vi "Drive at Angle.vi"(4 "end power":dbl, 6 "Begin power":dbl, 8 "error in (no error)":errorcluster, 9 "Angle":dbl, 10 "Distance":dbl, 11 "RobotDriveDevRef":T1={"DevStatus"={"status"=FALSE, "code"=0, "source"=""}, "Motors[]"=[], "Square Inputs"=FALSE, "Max Output"=1.0}) -> (0 "error out":errorcluster, 1 "power out":dbl, 3 "refnum":T1={"DevStatus"={"status"=FALSE, "code"=0, "source"=""}, "Motors[]"=[], "Square Inputs"=FALSE, "Max Output"=1.0})   [LabVIEW 2017]
uses:
  <vilib>/Rock Robotics/WPI/RobotDrive/WPI_RobotDriveDevRef.ctl
  <vilib>/Rock Robotics/WPI/MotorControl/WPI_MotorControlDeviceRef.ctl
  <vilib>/Rock Robotics/WPI/MotorControl/WPI_MotorControlType.ctl
  <vilib>/Rock Robotics/SystemInterfaces/DIO/FPGA_DIOPWMChannel.ctl
  <vilib>/Rock Robotics/WPI/PWM/WPI_PWMDeadband.ctl
  <vilib>/Rock Robotics/SystemInterfaces/DIO/FPGA_DIOChannel.ctl
  Robot Global Data.vi
  <vilib>/Rock Robotics/WPI/RobotDrive/WPI_RobotDriveArcadeDrive_Standard(NoSaturation).vi
panel:
  out "error":dbl
  out "x/y":dbl
  out "Distance Left 2":dbl format="%#_13g"
  out "rampdown":dbl format="%#_13g"
  out "Maximup":dbl format="%#_13g"
  out "rampup":dbl format="%#_13g"
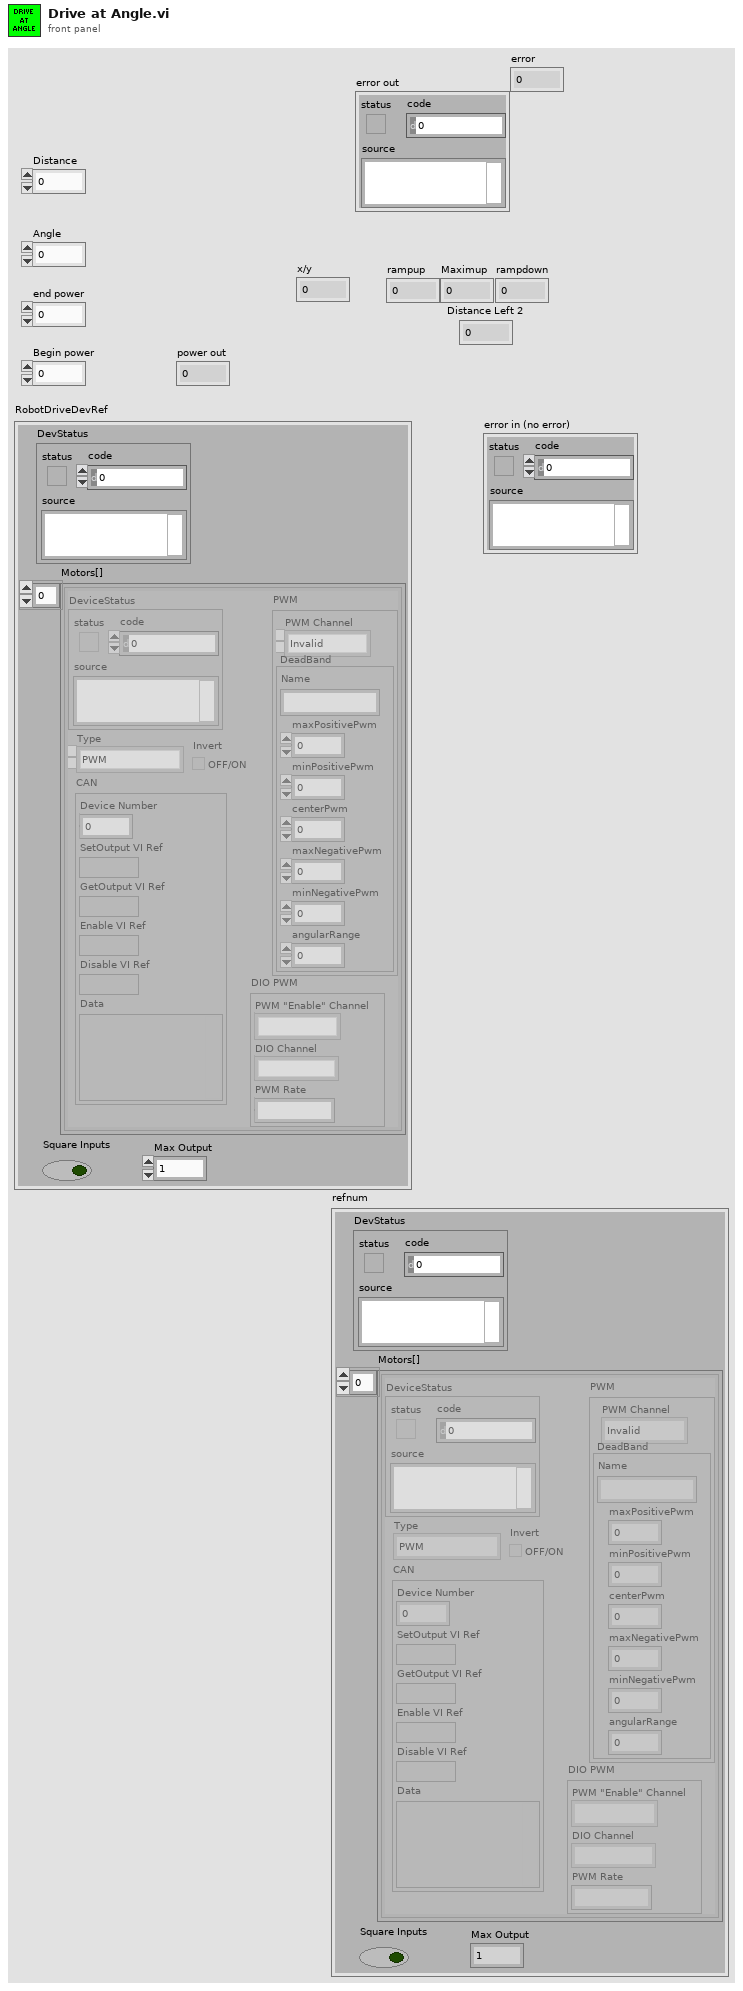
[diagram p1: front panel]
types:
  T1 = typedef "WPI_RobotDriveDevRef.ctl" = cluster{"DevStatus":errorcluster, "Motors[]":T2[], "Square Inputs":bool, "Max Output":dbl}
  T2 = typedef "WPI_MotorControlDeviceRef.ctl" = cluster{"DeviceStatus":errorcluster, "Type":T3, "PWM":cluster{"PWM Channel":T4, "DeadBand":T5}, "CAN":cluster{"Device Number":u8, "SetOutput VI Ref":variant, "GetOutput VI Ref":variant, "Enable VI Ref":variant, "Disable VI Ref":variant, "Data":variant}, "Invert":bool, "DIO PWM":cluster{"PWM \"Enable\" Channel":T4, "DIOChannel":T6, "PWM Rate":dbl}}
  T3 = typedef "WPI_MotorControlType.ctl" = enum16{"PWM", "CAN", "DIO PWM"}
  T4 = typedef "FPGA_DIOPWMChannel.ctl" = enum8{"PWM 0", "PWM 1", "PWM 2", "PWM 3", "PWM 4", "PWM 5", "PWM 6", "PWM 7", "PWM 8", "PWM 9", "PWM MXP 0", "PWM MXP 1", "PWM MXP 2", "PWM MXP 3", "PWM MXP 4", "PWM MXP 5", "PWM MXP 6", "PWM MXP 7", "PWM MXP 8", "PWM MXP 9", "Invalid"}
  T5 = typedef "WPI_PWMDeadband.ctl" = cluster{"Name":string, "maxPositivePwm":i32, "minPositivePwm":i32, "centerPwm":i32, "maxNegativePwm":i32, "minNegativePwm":i32, "angularRange":u16}
  T6 = typedef "FPGA_DIOChannel.ctl" = enum8{"DIO 0", "DIO 1", "DIO 2", "DIO 3", "DIO 4", "DIO 5", "DIO 6", "DIO 7", "DIO 8", "DIO 9", "DIO MXP 0", "DIO MXP 1", "DIO MXP 2", "DIO MXP 3", "DIO MXP 4", "DIO MXP 5", "DIO MXP 6", "DIO MXP 7", "DIO MXP 8", "DIO MXP 9", "DIO MXP 10", "DIO MXP 11", "DIO MXP 12", "DIO MXP 13", "DIO MXP 14", "DIO MXP 15", "SPI Port CS1", "SPI Port CS2", "SPI Port CS3", "SPI Port MISO", "SPI Port MOSI", "Invalid"}
  T7 = typedef "WPI_EncoderDevRef.ctl" = cluster{"DevStatus":errorcluster, "EncoderIndex":T8, "CounterIndex":T9, "DistancePerCount":dbl, "Decoding Type":T10}
  T8 = typedef "FPGA_EncoderIdx.ctl" = enum8{"Enc 0", "Enc 1", "Enc 2", "Enc 3", "Enc 4", "Enc 5", "Enc 6", "Enc 7", "Invalid"}
  T9 = typedef "FPGA_CounterCtrSystemIndex.ctl" = enum8{"Ctr 0", "Ctr 1", "Ctr 2", "Ctr 3", "Ctr 4", "Ctr 5", "Ctr 6", "Ctr 7", "Invalid"}
  T10 = typedef "WPI_EncoderType.ctl" = enum16{"1x", "2x", "4x"}
  T11 = cluster{"Yaw":dbl, "Roll":dbl, "Pitch":dbl, "Heading":dbl, "Fused Heading":dbl}
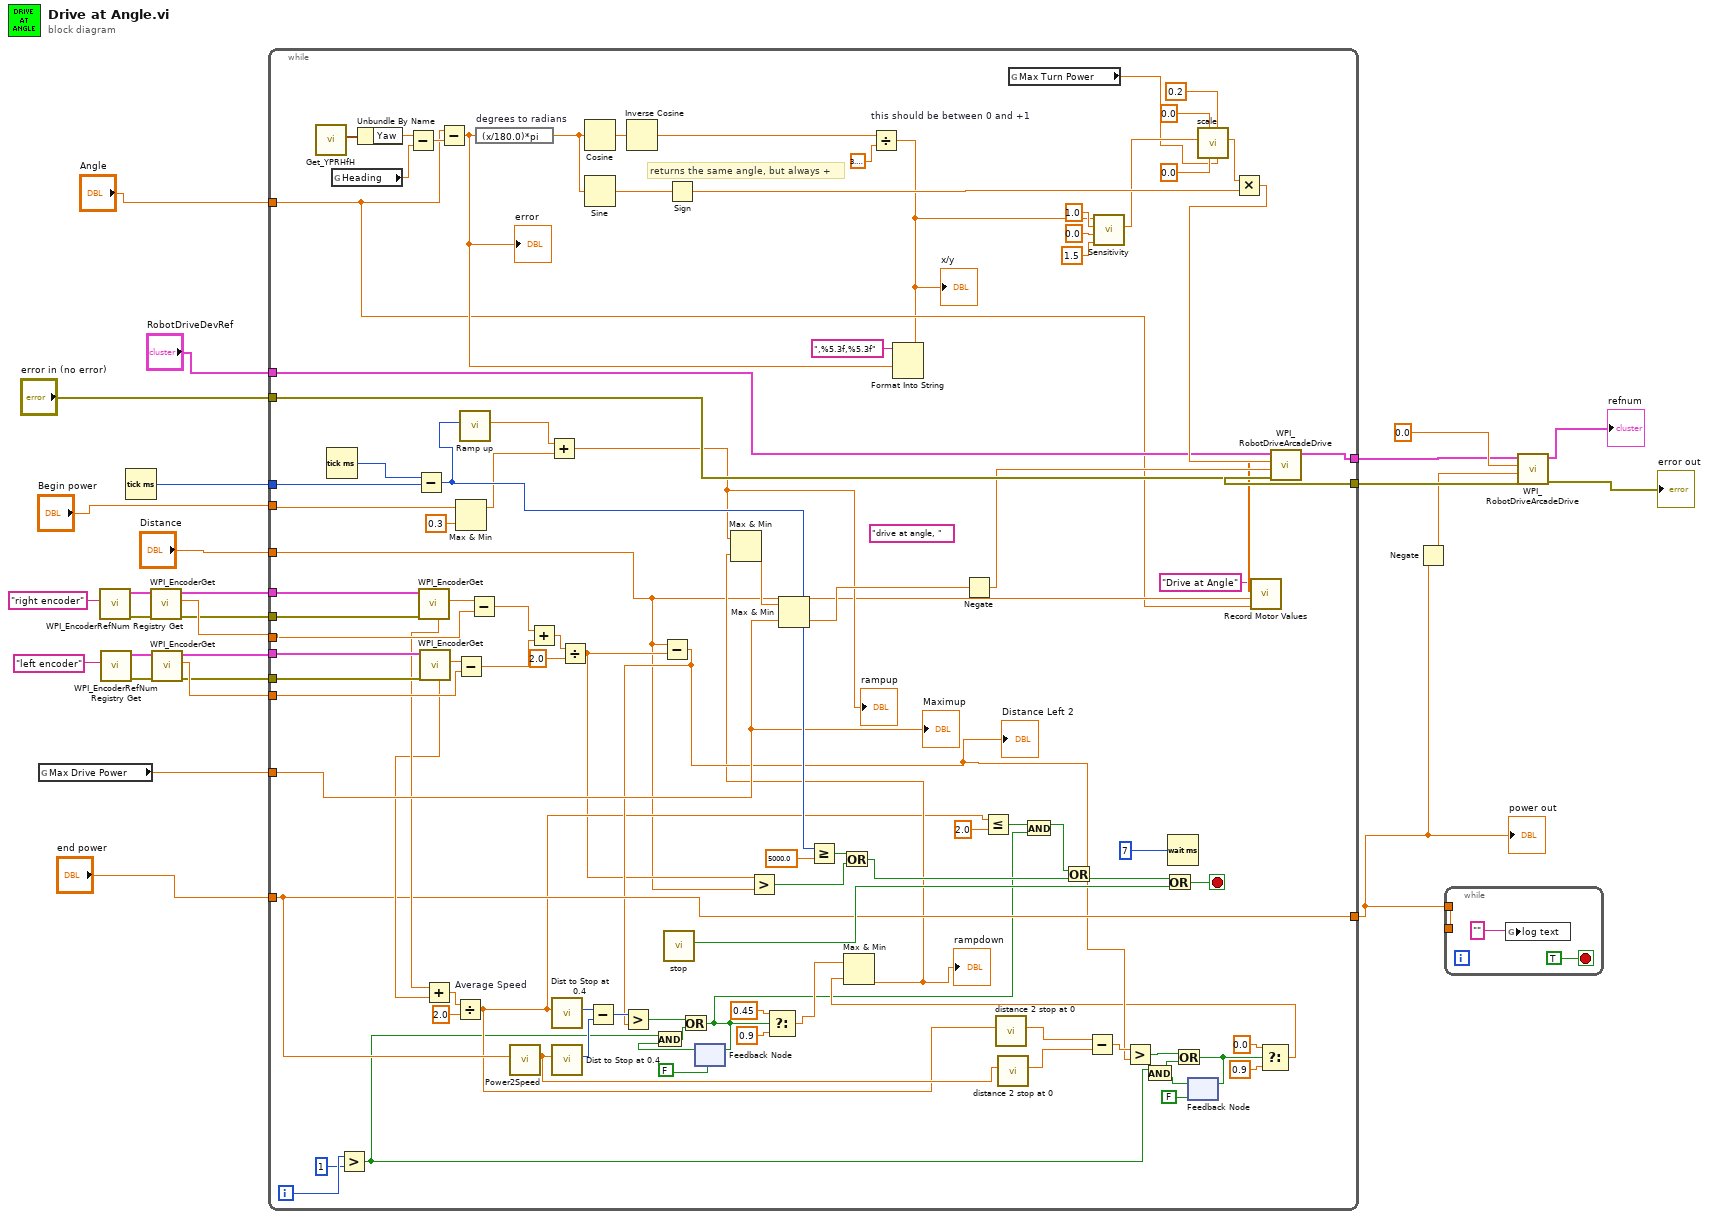
[diagram p0: block diagram]
diagram:
  n1 = global read "Robot Global Data.vi" "Max Drive Power"() -> (w3:dbl)
  n2 = call <vilib>:"WPI_EncoderRefNum Registry Get.vi"("refnum name"="right encoder") -> ("error out"=w27:errorcluster, "EncoderDevRef"=w26:T7)  [unwired: 9 in]
  n3 = call <vilib>:"WPI_EncoderRefNum Registry Get.vi"("refnum name"="left encoder") -> ("error out"=w24:errorcluster, "EncoderDevRef"=w23:T7)  [unwired: 9 in]
  n4 = Tick Count (ms)() -> (millisecond timer value=w12:u32)
  n5 = call <vilib>:"WPI_EncoderGet.vi"("error in (no error)"=w27, "EncoderDevRef"=w26) -> ("error out"=w15:errorcluster, "Distance"=w21:dbl, "EncoderDevRef"=w16:T7)  [unwired: 4 in, 3 out]
  n6 = call <vilib>:"WPI_EncoderGet.vi"("error in (no error)"=w24, "EncoderDevRef"=w23) -> ("error out"=w14:errorcluster, "Distance"=w20:dbl, "EncoderDevRef"=w13:T7)  [unwired: 4 in, 3 out]
  n7 = while {
    tunnel: "Distance" -> [w38]
    tunnel: w21 -> [w125]
    tunnel: w20 -> [w126]
    tunnel: [w124] -> w18
    tunnel: [w123] -> w17
    tunnel: w16 -> [w122]
    tunnel: w15 -> [w121]
    tunnel: w14 -> [w120]
    tunnel: w13 -> [w119]
    tunnel: w12 -> [w113]
    tunnel: [w78] -> w1
    tunnel: "Angle" -> [w37]
    tunnel: "end power" -> [w78]
    tunnel: "RobotDriveDevRef" -> [w89]
    tunnel: "error in (no error)" -> [w88]
    tunnel: "Begin power" -> [w35]
    tunnel: w3 -> [w83]
    i -> [w48]
    stop <- w91 stop-if-true
    (unwired) "drive at angle, " ("string")
    # "returns the same angle, but always +"
    n8 = call <vilib>:"Get_YPRHfH.vi"() -> ("YRPHfH"=w111:T11)  [unwired: 11 in]
    n9 = Tick Count (ms)() -> (millisecond timer value=w112:u32)
    n10 = global read "Robot Global Data.vi" "Heading"() -> (w106:dbl)
    n11 = Greater?(x=w48, y=1) -> (0:w44:bool)
    n12 = Unbundle By Name(w111) -> ("Yaw"=w107:dbl)
    n13 = Subtract(x=w107, y=w106) -> (x-y=w105:dbl)
    n14 = Subtract(x=w112, y=w113) -> (x-y=w90:u32)
    n15 = call <vilib>:"WPI_EncoderGet.vi"("error in (no error)"=w121, "EncoderDevRef"=w122) -> ("Distance"=w128:dbl, "Rate"=w80:dbl)  [unwired: 4 in, 4 out]
    n16 = call <vilib>:"WPI_EncoderGet.vi"("error in (no error)"=w120, "EncoderDevRef"=w119) -> ("Distance"=w127:dbl, "Rate"=w79:dbl)  [unwired: 4 in, 4 out]
    n17 = Add(x=w80, y=w79) -> (x+y=w81:dbl)
    n18 = Subtract(x=w37, y=w105) -> (x-y=w43:dbl)
    "error" <- w43
    n19 = Divide "Average Speed"(x=w81, y=2.0) -> (x/y=w52:dbl)
    n20 = Max & Min(x=w35, y=0.3) -> (max(x,y)=w36:dbl)  [unwired: 1 out]
    n21 = Subtract(x=w127, y=w126) -> (x-y=w115:dbl)
    n22 = call "Ramp up.vi"("time"=w90) -> ("Power Out"=w87:dbl)  [unwired: 10 in]
    n23 = Subtract(x=w128, y=w125) -> (x-y=w116:dbl)
    n24 = expression code="(x/180.0)*pi" "degrees to radians"(w43) -> (w108:dbl)
    n25 = call "Power2Speed.vi"("Power"=w78) -> ("Speed"=w67:dbl)  [unwired: 10 in]
    n26 = Add(x=w116, y=w115) -> (x+y=w118:dbl)
    n27 = Add(x=w87, y=w36) -> (x+y=w84:dbl)
    "rampup" <- w84
    n28 = call "Dist to Stop at 0.4.vi"("Speed"=w52) -> ("Distance"=w77:i32)  [unwired: 10 in]
    n29 = call "Dist to Stop at 0.4.vi"("Speed"=w67) -> ("Distance"=w76:i32)  [unwired: 10 in]
    n30 = Divide(x=w118, y=2.0) -> (x/y=w49:dbl)
    n31 = Cosine(x=w108) -> (cos(x)=w110:dbl)
    n32 = Sine(x=w108) -> (sin(x)=w109:dbl)
    n33 = Subtract(x=w77, y=w76) -> (x-y=w75:i32)
    n34 = Inverse Cosine(1:w110) -> (0:w103:dbl)
    n35 = Subtract(x=w38, y=w49) -> (x-y=w65:dbl)
    "Distance Left 2" <- w65
    n36 = Greater?(x=w75, y=w65) -> (0:w74:bool)
    n37 = call "stop.vi"() -> ("Boolean"=w93:bool)  [unwired: 11 in]
    n38 = Sign(1:w109) -> (0:w98:dbl)
    n39 = feedback #1(FALSE) -> (w73:bool)
    n40 = And(x=w44, y=w73) -> (x .and. y?=w46:bool)
    n41 = Or(x=w74, y=w46) -> (x .or. y?=w50:bool)
    n42 = feedback-in #1(w50) -> ()
    n43 = Greater?(x=w49, y=w38) -> (0:w94:bool)
    n44 = Select(t=0.45, s=w50, f=0.9) -> (s? t:f=w57:dbl)
    n45 = Greater Or Equal?(x=w90, y=5000.0) -> (x >= y?=w95:bool)
    n46 = Or(x=w95, y=w94) -> (x .or. y?=w92:bool)
    n47 = Divide "this should be between 0 and +1"(x=w103, y=3.141592653589793) -> (x/y=w30:dbl)
    "x/y" <- w30
    n48 = Format Into String(initial string=",%5.3f,%5.3f", w43, w30) -> ()  [unwired: 2 in, 2 out]
    n49 = Less Or Equal?(x=w52, y=2.0) -> (x <= y?=w54:bool)
    n50 = call "distance 2 stop at 0.vi"("speed"=w52) -> ("Distance"=w69:dbl)  [unwired: 10 in]
    n51 = call "distance 2 stop at 0.vi"("speed"=w67) -> ("Distance"=w68:dbl)  [unwired: 10 in]
    n52 = global read "Robot Global Data.vi" "Max Turn Power"() -> (w28:dbl)
    n53 = And(x=w54, y=w50) -> (x .and. y?=w51:bool)
    n54 = Or(x=w51, y=w92) -> (x .or. y?=w55:bool)
    n55 = Subtract(x=w69, y=w68) -> (x-y=w66:dbl)
    n56 = call "Sensitivity.vi"("Sensitivity"=1.5, "Low"=0.0, "High"=1.0, "Signal"=w30) -> ("Output"=w29:dbl)  [unwired: 7 in]
    n57 = Greater?(x=w66, y=w65) -> (0:w59:bool)
    n58 = Or(x=w55, y=w93) -> (x .or. y?=w91:bool)
    n59 = Wait (ms)(milliseconds to wait=u32 7) -> ()  [unwired: 1 out]
    n60 = feedback #2(FALSE) -> (w63:bool)
    n61 = And(x=w44, y=w63) -> (x .and. y?=w45:bool)
    n62 = Or(x=w59, y=w45) -> (x .or. y?=w64:bool)
    n63 = feedback-in #2(w64) -> ()
    n64 = call "scale.vi"("Max"=w28, "High"=0.2, "Min"=0.0, "Low"=0.0, "In Signal"=w29) -> ("Output signal"=w99:dbl)  [unwired: 6 in]
    n65 = Multiply(x=w99, y=w98) -> (x*y=w97:dbl)
    n66 = Select(t=0.0, s=w64, f=0.9) -> (s? t:f=w58:dbl)
    n67 = Max & Min(x=w57, y=w58) -> (min(x,y)=w56:dbl)  [unwired: 1 out]
    "rampdown" <- w56
    n68 = Max & Min(x=w84, y=w56) -> (min(x,y)=w86:dbl)  [unwired: 1 out]
    n69 = Max & Min(x=w86, y=w83) -> (min(x,y)=w85:dbl)  [unwired: 1 out]
    n70 = Negate(x=w85) -> (-x=w41:dbl)
    n71 = call-poly <vilib>:"WPI_RobotDriveArcadeDrive.vi"("error in (no error)"=w88, "Y axis value"=w41, "X axis value"=w97, "RobotDriveDevRef"=w89) -> ("error out"=w124:errorcluster, "Motor Values"=w40:dbl[], "RobotDriveDevRef"=w123:T1)  [unwired: 5 out]
    n72 = call "Record Motor Values.vi"("Target1 2"=w37, "Target1"=w38, "Motor Values"=w40, "VI Block Name"="Drive at Angle") -> ()  [unwired: 8 in]
    "Maximup" <- w83
  }
  "power out" <- w1
  n73 = Negate(x=w1) -> (-x=w2:dbl)
  n74 = while {
    tunnel: [w131] -> _
    tunnel: w1 -> [w131]
    stop <- TRUE stop-if-true
    n75 = global write "Robot Global Data.vi" "log text"("") -> ()
  }
  n76 = call-poly <vilib>:"WPI_RobotDriveArcadeDrive.vi"("error in (no error)"=w18, "Y axis value"=w2, "X axis value"=0.0, "RobotDriveDevRef"=w17) -> ("error out"=→"error out":errorcluster, "RobotDriveDevRef"=→"refnum":T1)  [unwired: 6 out]
